vi "Identify Obstacles.vi"(9 "filtered indices":i32[](array[numeric]), 10 "Filtered Slopes":dbl[](array[numeric]), 11 "window size":i32=4) -> (3 "Array 2":i32[](array[numeric]))   [LabVIEW 2017]
panel:
  out "Array":bool[](array[boolean])
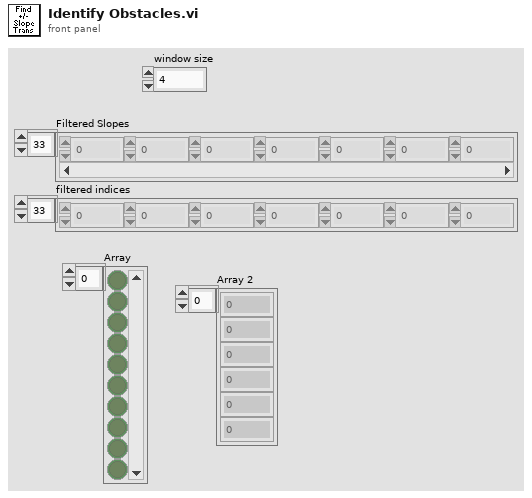
[diagram p1: front panel]
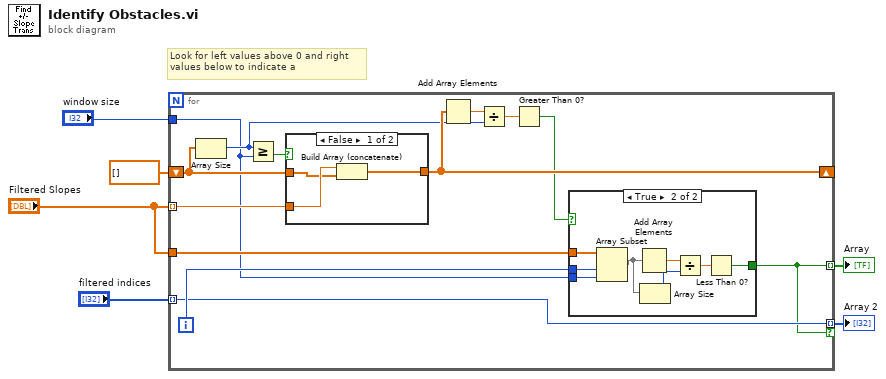
[diagram p0: block diagram]
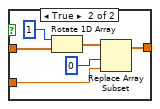
[diagram p3: hidden frame]
diagram:
  # "Look for left values above 0 and right\nvalues below to indicate a"
  n1 = for {
    tunnel: "Filtered Slopes" -> [w19] mode=indexing
    shift-right: [w16] -> _
    shift-left: dbl[] [] -> [w18]
    tunnel: "window size" -> [w9]
    tunnel: "Filtered Slopes" -> [w11]
    tunnel: [w7] -> w3 mode=indexing
    tunnel: [w8] -> w1 mode=indexing if=w7
    tunnel: "filtered indices" -> [w8] mode=indexing
    i -> [w10]
    n2 = Array Size(array=w18) -> (size(s)=w14:i32)
    n3 = Greater Or Equal?(x=w14, y=w9) -> (x >= y?=w17:bool)
    n4 = case shown="False" w17 {
      tunnel: w18 -> [w28 w36]
      tunnel: w19 -> [w29 w34]
      tunnel: [w30 w32] -> w16
      frame False {
        n5 = Build Array (concatenate)(w29, w28) -> (w30:dbl[])
      }
      frame True {
        n6 = Rotate 1D Array(1:w36, 2:1 ("n")) -> (0:w35:dbl[])
        n7 = Replace Array Subset(array=w35, new element=w34, index=0) -> (w32:dbl[])
      }
    }
    n8 = Add Array Elements(numeric array=w16) -> (sum=w15:dbl)
    n9 = Divide(x=w15, y=w14) -> (x/y=w13:dbl)
    n10 = Greater Than 0?(x=w13) -> (x > 0?=w12:bool)
    n11 = case shown="True" w12 {
      tunnel: w11 -> [_ w27]
      tunnel: w10 -> [_ w26]
      tunnel: w9 -> [_ w25]
      tunnel: [_ w20] -> w7
      frame False {
      }
      frame True {
        n12 = Array Subset(array=w27, index=w26, length=w25) -> (w23:dbl[])
        n13 = Add Array Elements(numeric array=w23) -> (sum=w24:dbl)
        n14 = Array Size(array=w23) -> (size(s)=w22:i32)
        n15 = Divide(x=w24, y=w22) -> (x/y=w21:dbl)
        n16 = Less Than 0?(x=w21) -> (x < 0?=w20:bool)
      }
    }
  }
  "Array" <- w3
  "Array 2" <- w1
